vi "libssh2_channel_free.vi"(8 "error in (no error)":errorcluster, 11 "channel":T1) -> (0 "error out":errorcluster)   [LabVIEW 2013, in "libssh2.lvlib"]
doc: "Frees all resouces associated with a channel."
uses:
  libssh2.lvlib
  Channel Refnum.ctl
  Global Settings.vi
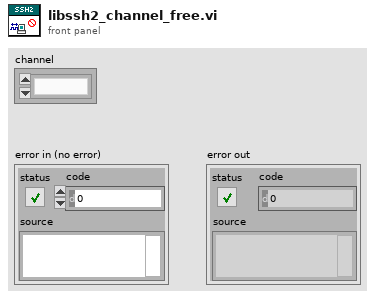
[diagram p1: front panel]
types:
  T1 = typedef "libssh2.lvlib/Channel Refnum.ctl" = refnum<k1>
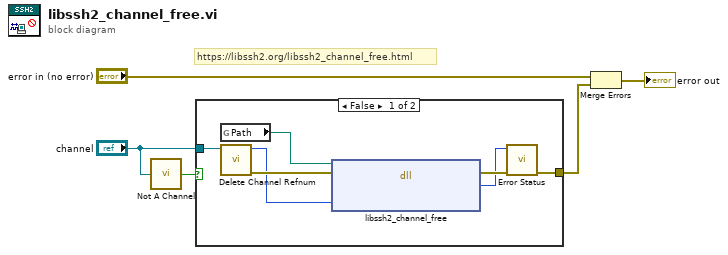
[diagram p0: block diagram]
diagram:
  # "https://libssh2.org/libssh2_channel_free.html"
  n1 = call "Not A Channel.vi"("channel"="channel") -> ("Not a Channel?"=w1:bool)
  n2 = case shown="False" w1 {
    tunnel: "channel" -> [w10 _]
    tunnel: [w7 _] -> w5
    frame False {
      n3 = global read "Global Settings.vi" "Path"() -> (w8:path)
      n4 = call "Delete Channel Refnum.vi"("channel"=w10) -> ("error out"=w12:errorcluster, "LIBSSH2_CHANNEL*"=w11:u64)  [unwired: 9 in]
      n5 = dll-call lib="C:/Users/pasca/source/repos/libssh2-labview/libssh2/libssh2**.*" fn="libssh2_channel_free"(path in=w8, error in=w12, "channel"=w11) -> (error out=w9:errorcluster, "return value"=w6:i32)  [unwired: 2 in, 1 out]
      n6 = call "Error Status.vi"("error in (no error)"=w9, "return value"=w6) -> ("error out"=w7:errorcluster)  [unwired: 8 in, 1 out]
    }
    frame True {
    }
  }
  n7 = Merge Errors("error in (no error)", w5) -> (→"error out":errorcluster)
